vi "Init Spec Page.vi"(8 "error in (no error)":errorcluster, 9 "Wizard Interface":T1, 11 "MetaDataObj":refnum<class "MetaDataObj.lvclass">) -> (2 "VI Ref Out":refnum<vi>, 3 "SpecPage out":refnum<class "BaseSpecPage.lvclass">, 4 "SpecPage Ctrl #n Ref":refnum<vi>, 6 "SpecPage Ctrl #1 Ref":refnum<vi>)   [LabVIEW 2016]
uses:
  <resource>/dialog/NewProjectWizard/MetaDataObj/MetaDataObj.lvclass
  <resource>/dialog/NewProjectWizard/Spec Page Interface.ctl
  <resource>/dialog/NewProjectWizard/SpecPage/Base/BaseSpecPage.lvclass
  <resource>/dialog/NewProjectWizard/SpecPage/ConfirmQuitSpecPage/ConfirmQuitSpecPage.lvclass
  e:/builds/penguin/labview/branches/2016/dev/dist/resource/dialog/NewProjectWizard/SpecPage/Base/BaseSpecPage.lvclass
  <resource>/dialog/NewProjectWizard/MetaDataObj/Accessors/Read Hide Icon Overlay.vi
  <resource>/dialog/NewProjectWizard/MetaDataObj/Accessors/Read Hide Prefix.vi
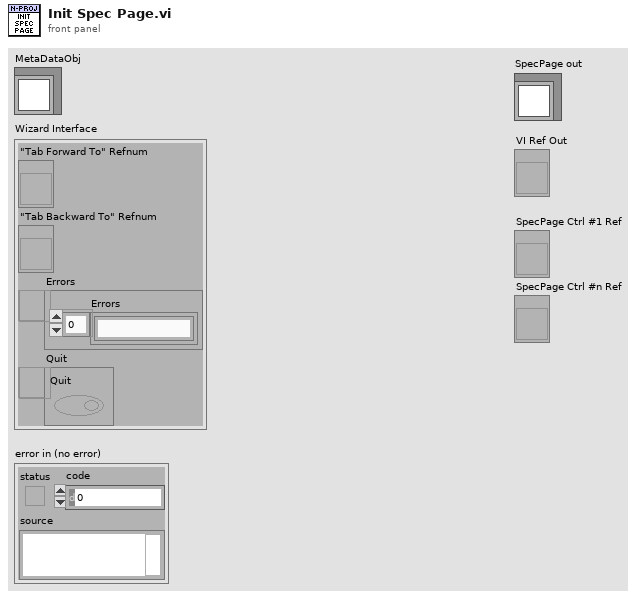
[diagram p1: front panel]
types:
  T1 = typedef "Spec Page Interface.ctl" = cluster{"\"Tab Forward To\" Refnum":refnum<vi>, "\"Tab Backward To\" Refnum":refnum<vi>, "Errors":refnum<user-event>, "Quit":refnum<user-event>}
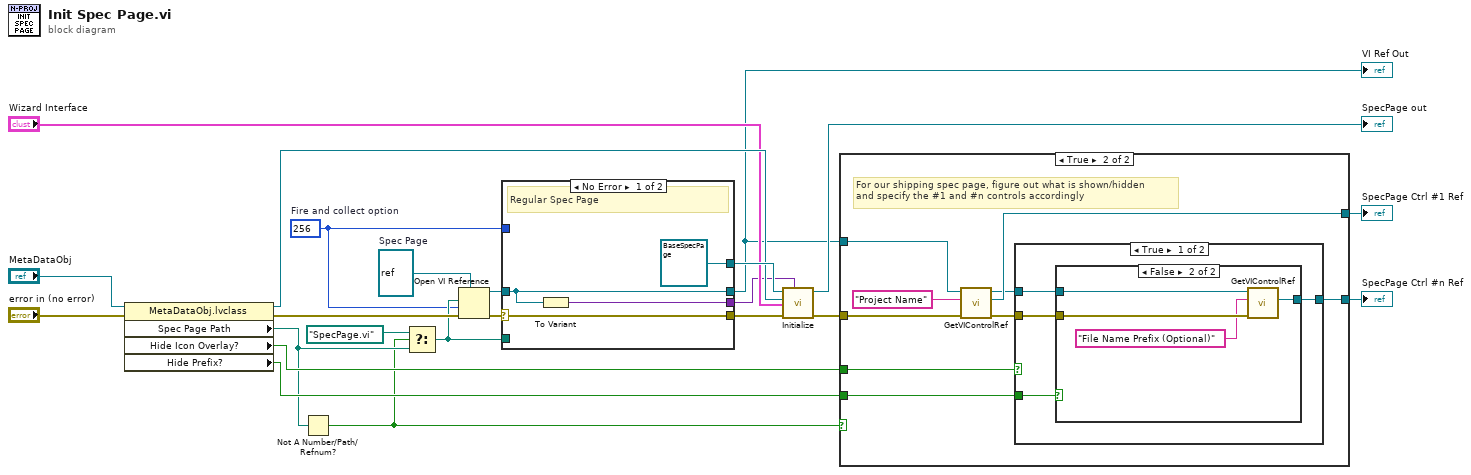
[diagram p0: block diagram]
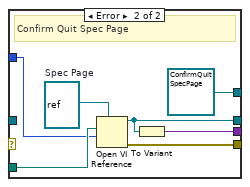
[diagram p2: hidden frame]
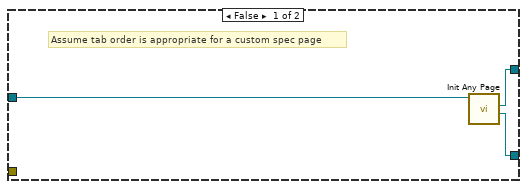
[diagram p3: hidden frame]
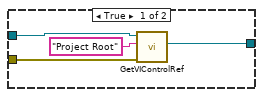
[diagram p4: hidden frame]
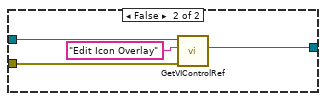
[diagram p5: hidden frame]
diagram:
  w19 = refnum<vi> refnum  # Spec Page
  w7 = 256  # Fire and collect option
  n1 = property class="MetaDataObj.lvclass"(reference="MetaDataObj", error in="error in (no error)") -> (reference out=w12:refnum<class "MetaDataObj.lvclass">, error out=w17:errorcluster, "Spec Page Path"=w2:path, "Hide Icon Overlay?"=w15:bool, "Hide Prefix?"=w14:bool)
  n2 = Not A Number/Path/Refnum?(number/path/refnum=w2) -> (NaN/Path/Refnum?=w1:bool)
  n3 = Select(t=path "SpecPage.vi", s=w1, f=w2) -> (s? t:f=w8:path)
  n4 = Open VI Reference(type specifier VI Refnum (for type only)=w19, vi path=w8, options=w7, error in (no error)=w17) -> (vi reference=w16:refnum<vi>, error out=w9:errorcluster)  [unwired: 2 in]
  n5 = case shown="No Error" w9 {
    selector: w9 -> [w26 _]
    tunnel: [w26 w33] -> w6
    tunnel: w16 -> [w25 _]
    tunnel: [w25 w29] -> w3
    tunnel: [refnum<class "BaseSpecPage.lvclass"> refnum ("BaseSpecPage in") refnum<class "ConfirmQuitSpecPage.lvclass"> refnum ("ConfirmQuitSpecPage.lvclass")] -> w13
    tunnel: w8 -> [_ w32]
    tunnel: w7 -> [_ w31]
    tunnel: [w24 w28] -> w4
    frame No Error {
      # "Regular Spec Page"
      n6 = To Variant(anything=w25) -> (Variant=w24:variant)
    }
    frame Error {
      w34 = refnum<vi> refnum  # Spec Page
      # "Confirm Quit Spec Page"
      n7 = Open VI Reference(type specifier VI Refnum (for type only)=w34, vi path=w32, options=w31) -> (vi reference=w29:refnum<vi>, error out=w33:errorcluster)  [unwired: 3 in]
      n8 = To Variant(anything=w29) -> (Variant=w28:variant)
    }
  }
  "VI Ref Out" <- w3
  n9 = call-dynamic "Initialize.vi"("VI Ref"=w4, "error in (no error)"=w6, "Wizard Interface"="Wizard Interface", "MetaDataObj in"=w12, "BaseSpecPage in"=w13) -> ("error out"=w5:errorcluster, "BaseSpecPage out"=→"SpecPage out":refnum<class "BaseSpecPage.lvclass">)  [unwired: 5 in]
  n10 = case shown="True" w1 {
    tunnel: [w37 w43] -> w21
    tunnel: [w36 w38] -> w20
    tunnel: w3 -> [w35 w45]
    tunnel: w5 -> [_ w46]
    tunnel: w15 -> [_ w40]
    tunnel: w14 -> [_ w39]
    frame False {
      # "Assume tab order is appropriate for a custom spec page"
      n11 = call <resource>:"Init Any Page.vi"("VI in"=w35) -> ("Page Ctrl #N Ref"=w36:refnum<vi>, "Page Ctrl #1 Ref"=w37:refnum<vi>)  [unwired: 9 in]
    }
    frame True {
      # "For our shipping spec page, figure out what is shown/hidden\nand specify the #1 and #n controls accordingly"
      n12 = call <resource>:"GetVIControlRef.vi"("error in"=w46, "Control Name"="Project Name", "VI Ref In"=w45) -> ("error out"=w41:errorcluster, "Control Reference"=w43:refnum<vi>, "VI Ref Out"=w42:refnum<vi>)  [unwired: 6 in]
      n13 = case shown="True" w40 {
        tunnel: w42 -> [w48 w61]
        tunnel: w41 -> [w49 w62]
        tunnel: w39 -> [w50 _]
        tunnel: [w47 w60] -> w38
        frame True {
          n14 = case shown="False" w50 {
            tunnel: w49 -> [w54 w58]
            tunnel: w48 -> [w53 w57]
            tunnel: [w52 w56] -> w47
            frame True {
              n15 = call <resource>:"GetVIControlRef.vi"("error in"=w54, "Control Name"="Project Root", "VI Ref In"=w53) -> ("Control Reference"=w52:refnum<vi>)  [unwired: 6 in, 2 out]
            }
            frame False {
              n16 = call <resource>:"GetVIControlRef.vi"("error in"=w58, "Control Name"="File Name Prefix (Optional)", "VI Ref In"=w57) -> ("Control Reference"=w56:refnum<vi>)  [unwired: 6 in, 2 out]
            }
          }
        }
        frame False {
          n17 = call <resource>:"GetVIControlRef.vi"("error in"=w62, "Control Name"="Edit Icon Overlay", "VI Ref In"=w61) -> ("Control Reference"=w60:refnum<vi>)  [unwired: 6 in, 2 out]
        }
      }
    }
  }
  "SpecPage Ctrl #1 Ref" <- w21
  "SpecPage Ctrl #n Ref" <- w20
